vi "Autocompleter.vi"() -> ()   [LabVIEW 2020]
doc: "This VI provides autocomplete suggestions for LabVIEW developers."
uses:
  Model/MarkovModel/MarkovModel.lvclass
  <vilib>/Utility/miscctls.llb/LVBoundsTypeDef.ctl
  <vilib>/Utility/miscctls.llb/LVPositionTypeDef.ctl
  <vilib>/Utility/miscctls.llb/LVPointTypeDef.ctl
panel:
  in  "Stop":bool
  in  "Autowire?":bool
  out "Suggested Block 4":picture caption="Option 4"
  out "Suggested Block 3":picture caption="Option 3"
  out "Suggested Block 2":picture caption="Option 2"
  out "Suggested Block 1":picture caption="Option 1"
  out "Position":T1
  out "Excluded?":bool
  out "Selected":string
  out "value":cluster{"Class Name":string, "Count":i32}[](array[cluster])
  out "One selected?":bool
  out "Active Window":u16(ring) items=["Front Panel", "Block Diagram"]
  out "Selected Object Types":string[](array[string])
  out "Selected VI":string
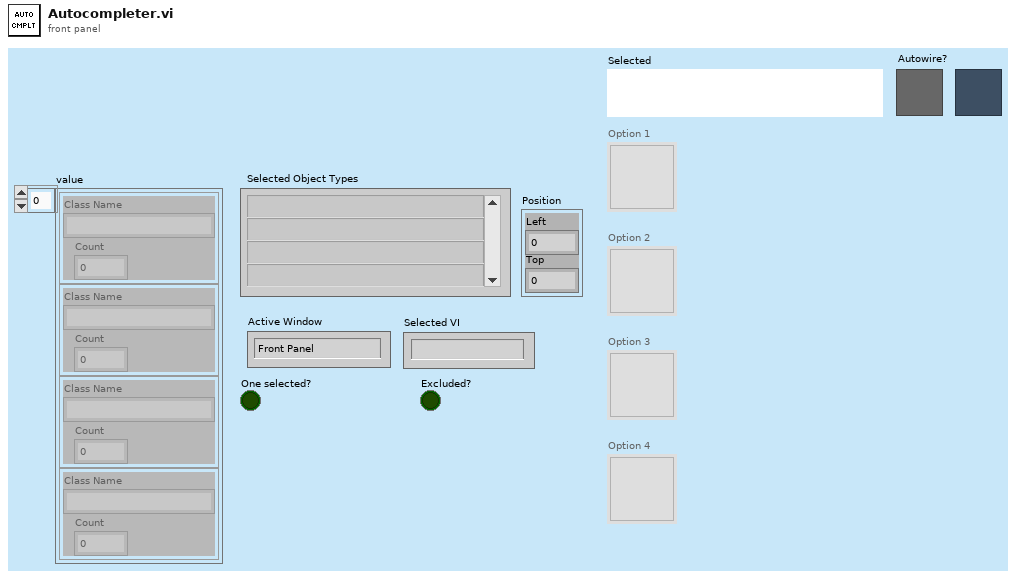
[diagram p1: front panel]
types:
  T1 = typedef "LVPositionTypeDef.ctl" = cluster{"Left":i32, "Top":i32}
  T2 = typedef "LVPointTypeDef.ctl" = cluster{"Horizontal":i16, "Vertical":i16}
  T3 = typedef "imagedata.ctl" = cluster{"image type":i32, "image depth":i32, "image":u8[], "mask":u8[], "colors":u32[], "Rectangle":cluster{"left":i16, "top":i16, "right":i16, "bottom":i16}}
  T4 = enum8{"Enabled", "Disabled", "Disabled and Grayed Out"}
  T5 = typedef "LVBoundsTypeDef.ctl" = cluster{"Width":u32, "Height":u32}
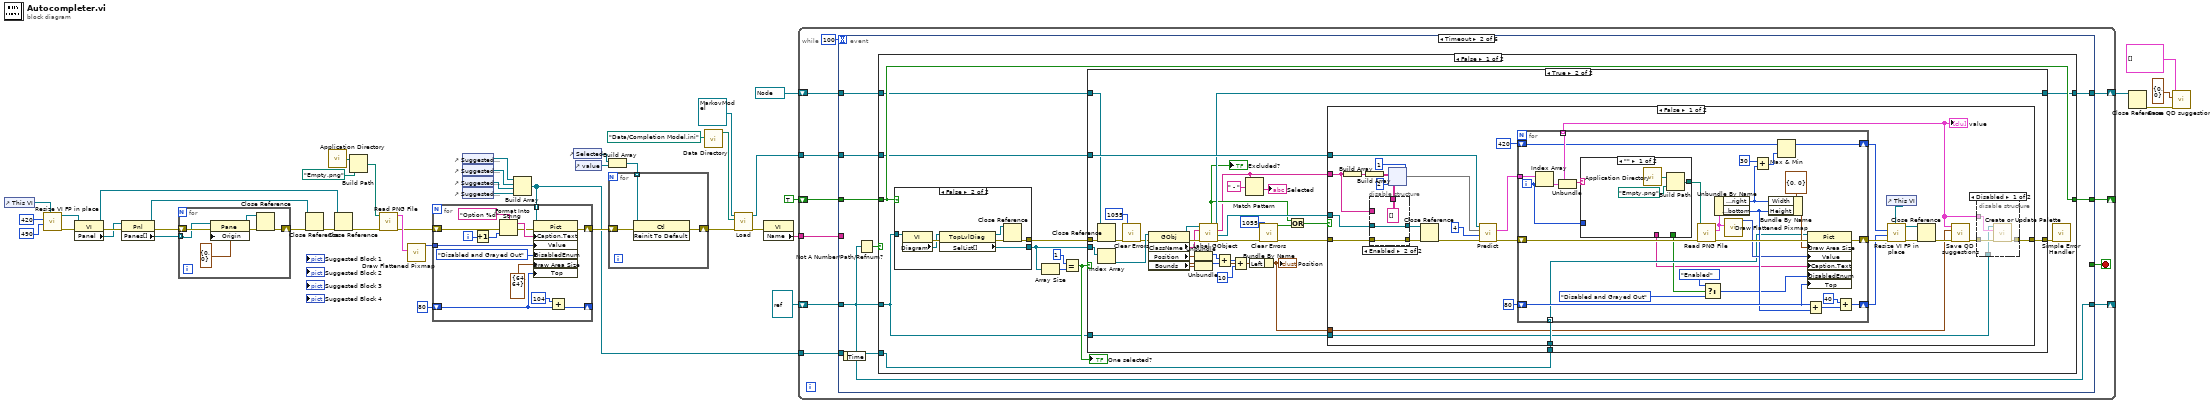
[diagram p0: block diagram]
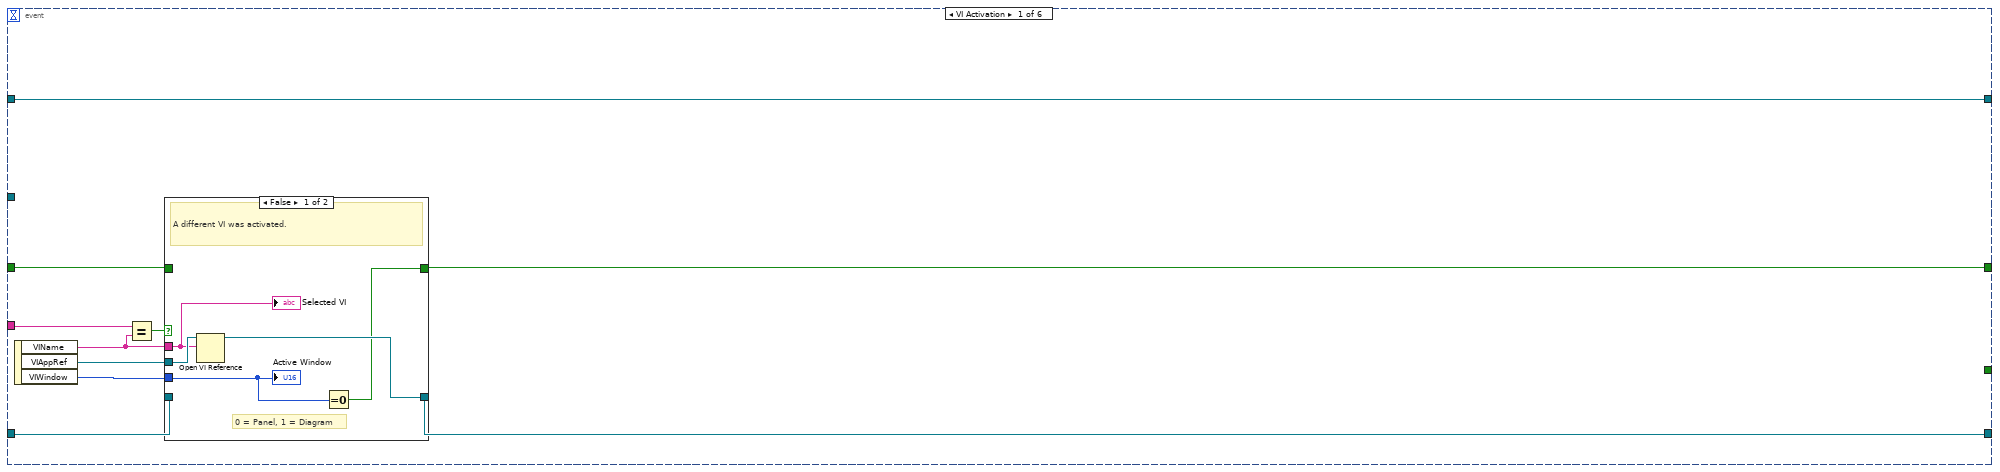
[diagram p2: hidden frame]
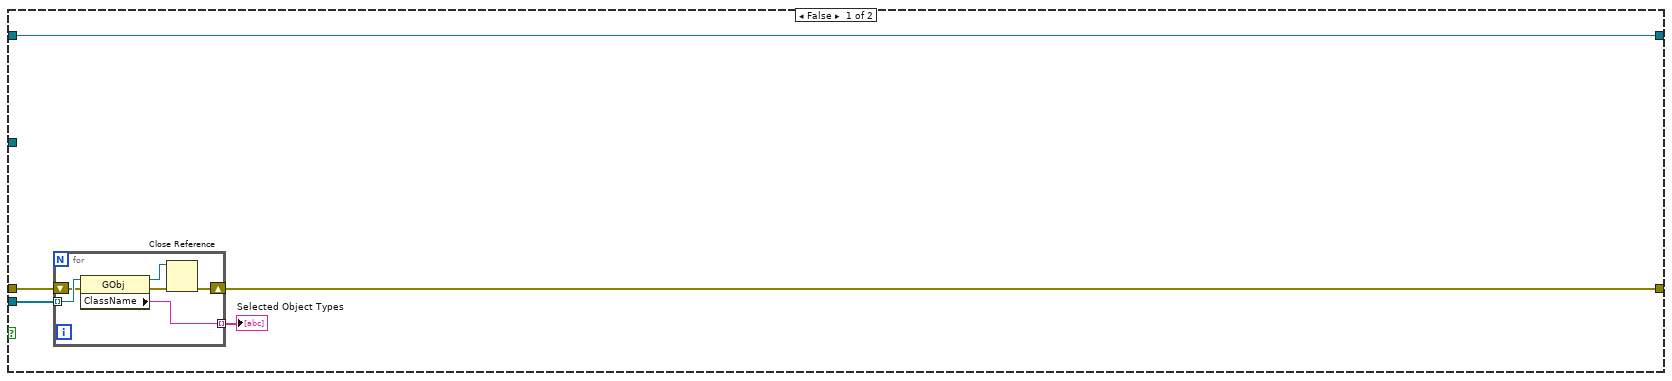
[diagram p4: hidden frame]
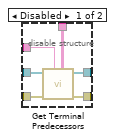
[diagram p6: hidden frame]
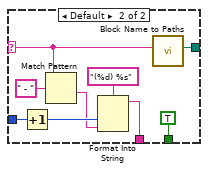
[diagram p7: hidden frame]
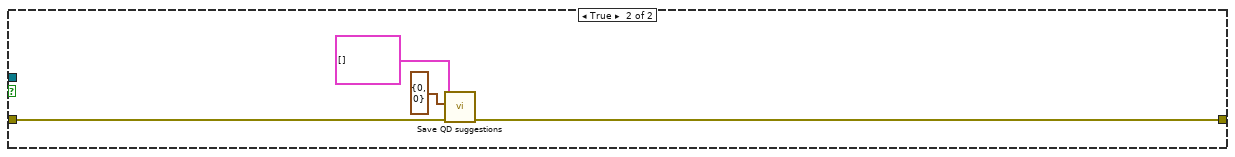
[diagram p8: hidden frame]
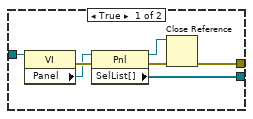
[diagram p9: hidden frame]
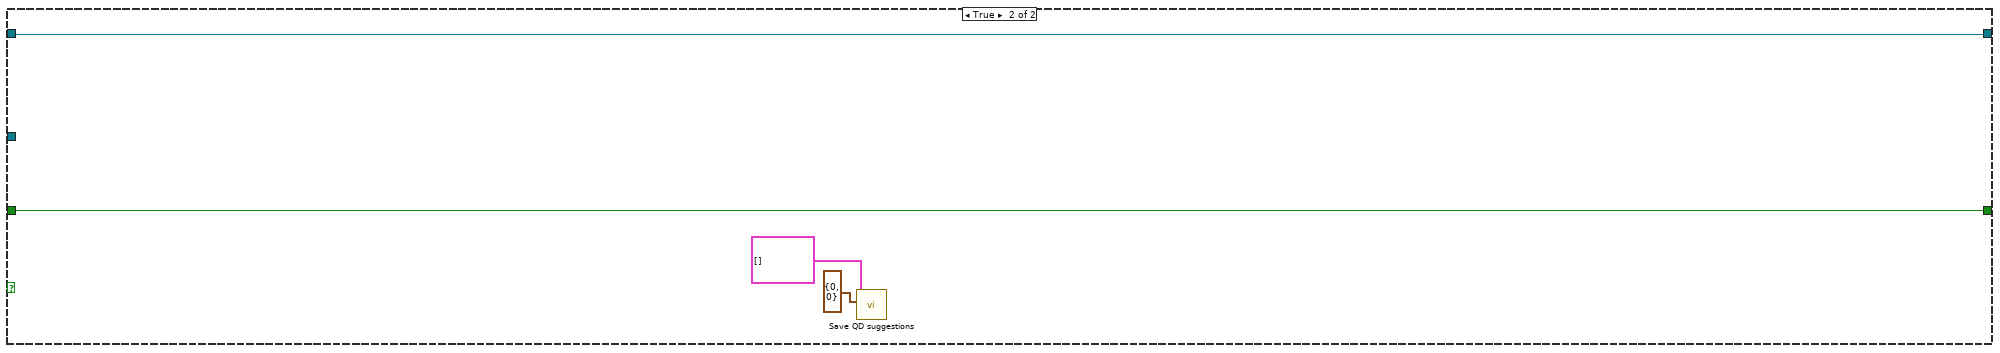
[diagram p10: hidden frame]
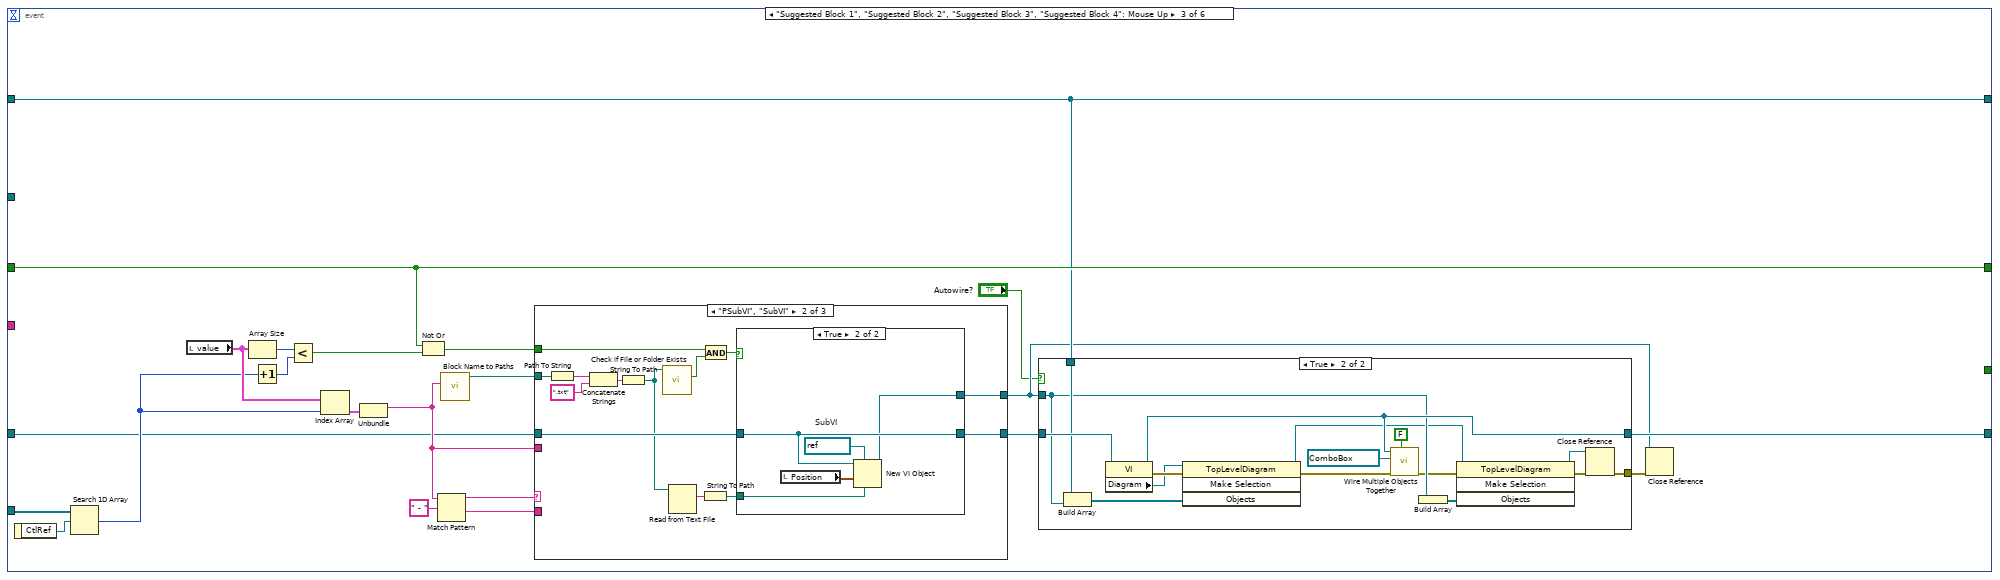
[diagram p11: hidden frame]
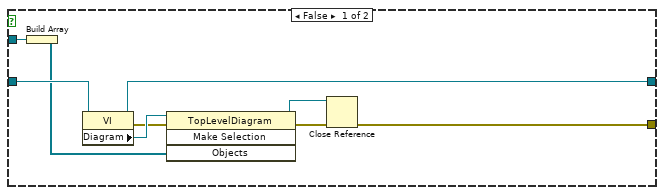
[diagram p12: hidden frame]
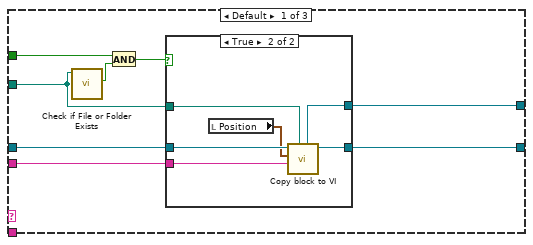
[diagram p13: hidden frame]
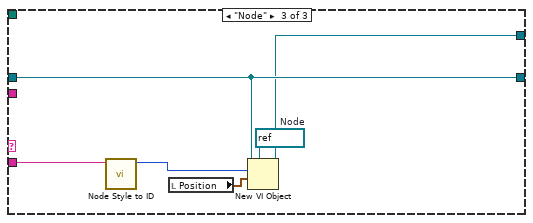
[diagram p16: hidden frame]
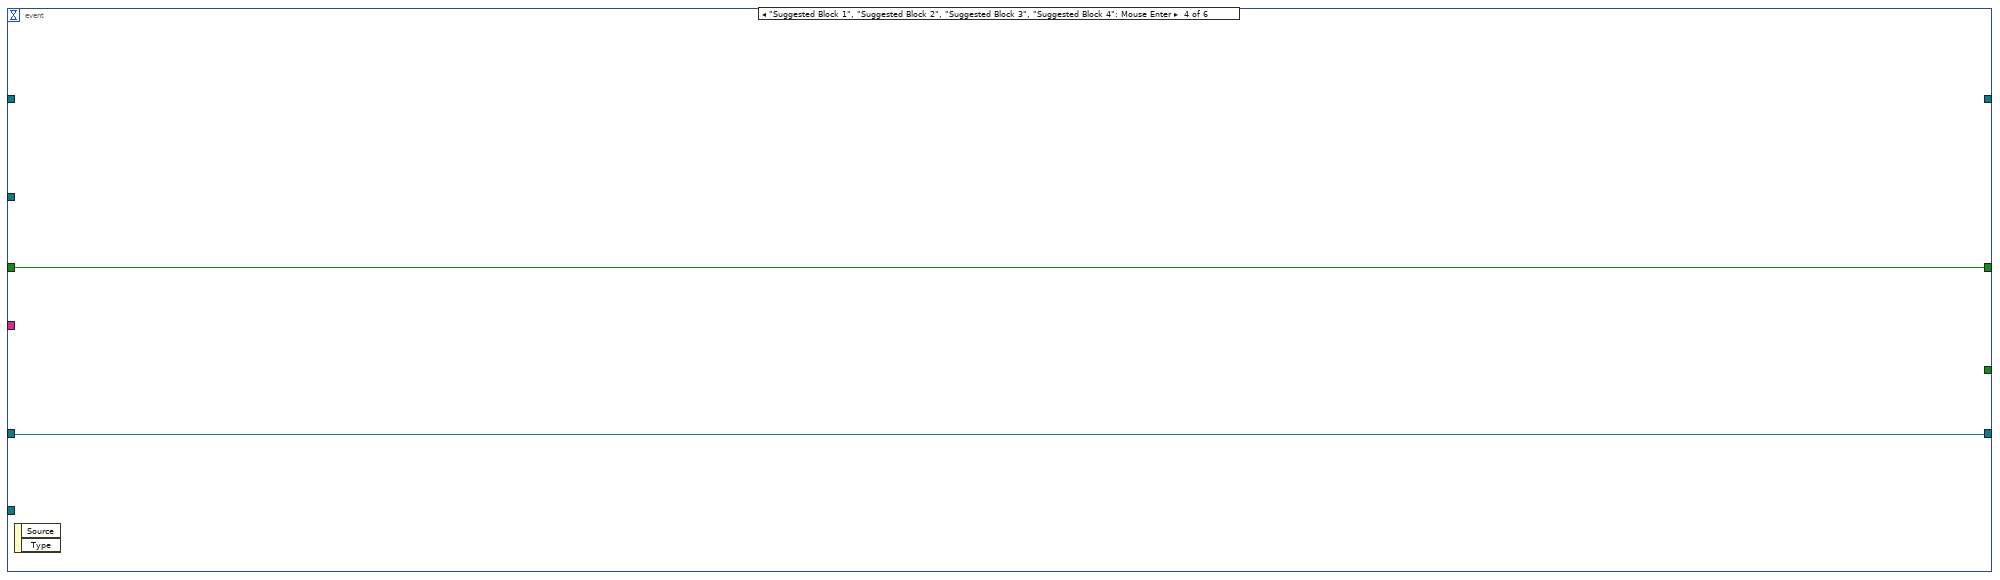
[diagram p17: hidden frame]
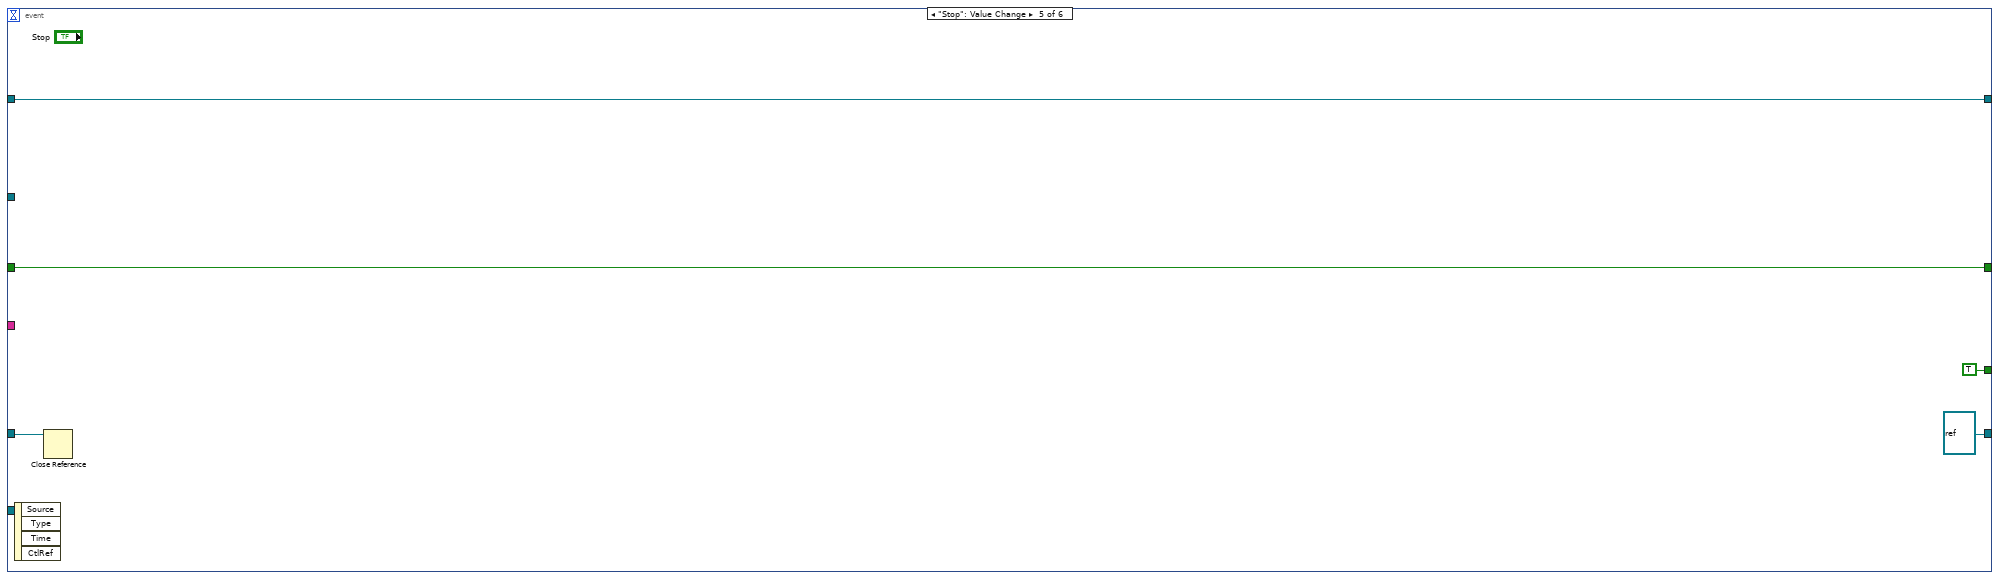
[diagram p18: hidden frame]
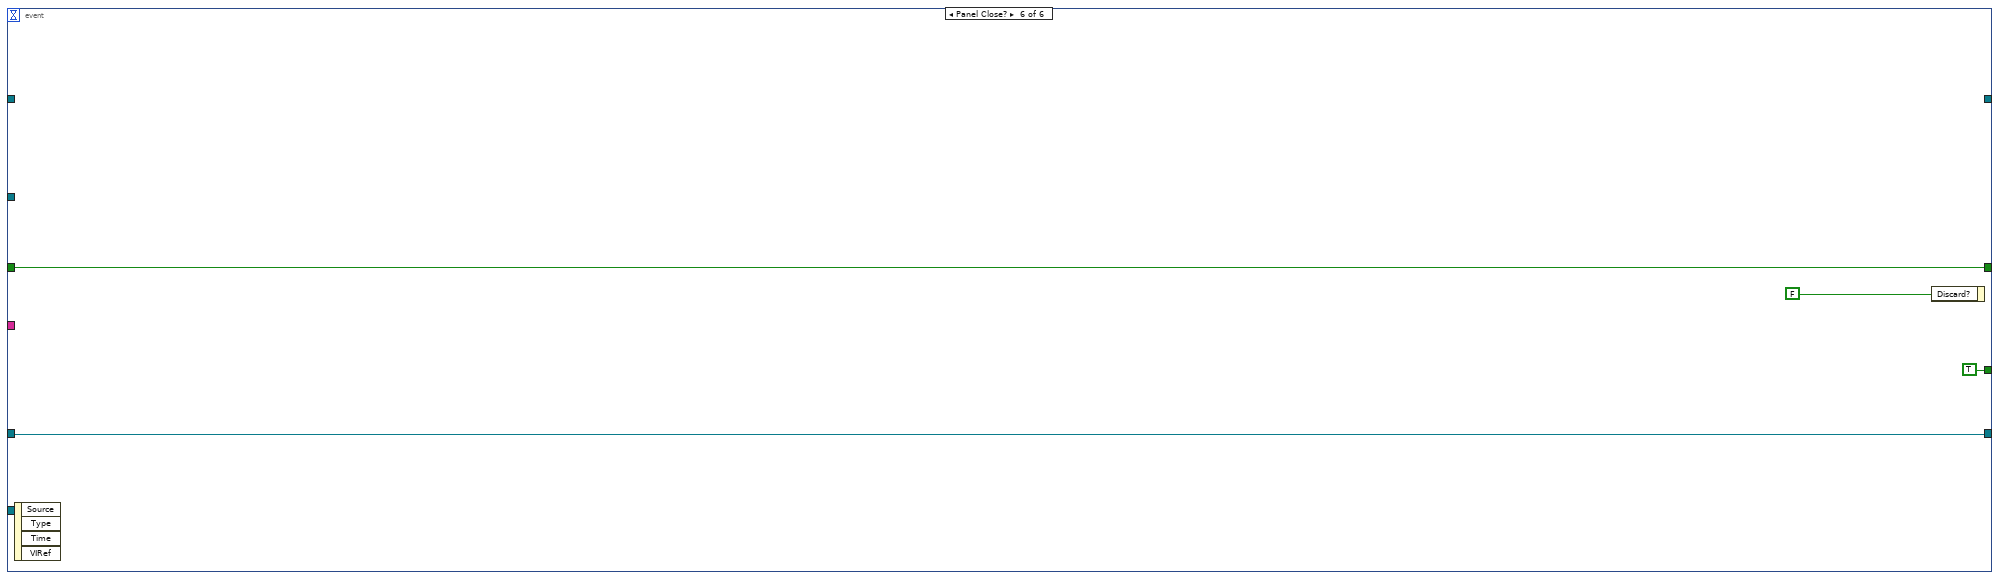
[diagram p19: hidden frame]
diagram:
  n1 = control-ref of="This VI"() -> (w19:refnum<vi>)
  n2 = call "Resize VI FP in place.vi"("VI reference in"=w19, "Height"=u32 490, "Width"=u32 420) -> ("error out"=w11:errorcluster, "VI reference out"=w8:refnum<vi>)  [unwired: 6 in, 1 out]
  n3 = property class="VI"(reference=w8, error in=w11) -> (reference out=w9:refnum<vi>, error out=w16:errorcluster, "Panel"=w7:refnum<vi>)
  n4 = property class="Pnl"(reference=w7, error in=w16) -> (reference out=w13:refnum<vi>, error out=w15:errorcluster, "Panes[]"=w12:refnum<vi>[])
  n5 = for {
    shift-right: [w46] -> w14
    shift-left: w15 -> [w50]
    tunnel: w12 -> [w45] mode=indexing
    n6 = property class="Pane"(reference=w45, error in=w50, "Origin"=T2 {"Horizontal"=0, "Vertical"=0}) -> (reference out=w47:refnum<vi>, error out=w48:errorcluster)
    n7 = Close Reference(reference=w47, error in (no error)=w48) -> (error out=w46:errorcluster)
  }
  n8 = Close Reference(reference=w13, error in (no error)=w14) -> (error out=w10:errorcluster)
  n9 = call <vilib>:"Application Directory.vi"() -> ("Application Directory"=w22:path)
  n10 = Close Reference(reference=w9, error in (no error)=w10) -> (error out=w20:errorcluster)
  n11 = Build Path(base path=w22, name or relative path=path "Empty.png") -> (appended path=w31:path)
  n12 = call <vilib>:"Read PNG File.vi"("error in (no error)"=w20, "path to PNG file"=w31) -> ("error out"=w30:errorcluster, "image data"=w32:T3)  [unwired: 7 in, 1 out]
  n13 = call <vilib>:"Draw Flattened Pixmap.vi"("image data"=w32) -> ("new picture"=w29:picture)  [unwired: 8 in]
  n14 = control-ref of="Suggested Block 1"() -> (w41:refnum<vi>)
  n15 = control-ref of="Suggested Block 2"() -> (w40:refnum<vi>)
  n16 = control-ref of="Suggested Block 3"() -> (w39:refnum<vi>)
  n17 = control-ref of="Suggested Block 4"() -> (w38:refnum<vi>)
  n18 = Build Array(w41, w40, w39, w38) -> (w21:refnum<vi>[])
  n19 = for {
    shift-right: [w64] -> w34
    shift-left: w30 -> [w60]
    tunnel: w21 -> [w63] mode=indexing
    tunnel: w29 -> [w58]
    shift-right: [w55] -> _
    shift-left: 80 -> [w57]
    i -> [w53]
    n20 = Increment(x=w53) -> (x+1=w52:i32)
    n21 = Format Into String(format string="Option %d", error in=w60, w52) -> (resulting string=w61:string, error out=w59:errorcluster)  [unwired: 1 in]
    n22 = property class="Pict"(reference=w63, error in=w59, "Caption.Text"=w61, "Value"=w58, "DisabledEnum"=T4."Disabled and Grayed Out" ("Disabled"), "Draw Area Size"=T5 {"Width"=64, "Height"=64}, "Top"=w57) -> (error out=w64:errorcluster)  [unwired: 1 out]
    n23 = Add(x=104, y=w57) -> (x+y=w55:i32)
  }
  n24 = control-ref of="Selected"() -> (w37:refnum<vi>)
  n25 = control-ref of="value"() -> (w36:refnum<vi>)
  n26 = Build Array(w37, w36) -> (w35:refnum<vi>[])
  n27 = for {
    shift-right: [w67] -> w5
    shift-left: w34 -> [w66]
    tunnel: w35 -> [w65] mode=indexing
    n28 = invoke on="Invoke Node" class="Ctl" method="Reinit To Default"(reference=w65, error in=w66) -> (error out=w67:errorcluster)  [unwired: 1 in, 2 out]
  }
  n29 = call "Data Directory.vi"("Subdirectory"=path "Data/Completion Model.ini" ("file (use dialog)")) -> ("Data directory"=w1:path)  [unwired: 9 in, 1 out]
  n30 = call-dynamic "Load.vi"("error in (no error)"=w5, "Model Path"=w1, "MarkovModel in"=refnum<class "MarkovModel.lvclass"> refnum ("MarkovModel.lvclass")) -> ("error out"=w4:errorcluster, "MarkovModel out"=w2:refnum<class "MarkovModel.lvclass">)  [unwired: 7 in]
  n31 = property class="VI"(error in=w4) -> ("Name"=w44:string)  [unwired: 1 in, 2 out]
  n32 = while {
    tunnel: w44 -> [w77]
    shift-right: [w76] -> _
    shift-left: refnum<vi> refnum ("VIAppRef") -> [w75]
    shift-right: [w72] -> _
    shift-left: TRUE -> [w73]
    tunnel: w2 -> [w71]
    tunnel: w21 -> [w70]
    shift-right: [w68] -> w26
    shift-left: refnum<vi> refnum ("element") -> [w69]
    stop <- w78 stop-if-true
    n33 = event shown="[1] Timeout" {
      selector: _ -> [_ _ _ _ _ _]
      dyn-events: _ -> [_ _ _ _ _ _]
      timeout: 100 -> [_ _ _ _ _ _]
      tunnel: [_ _ _ _ TRUE ("Stop") TRUE ("Stop")] -> w78
      tunnel: w77 -> [w87 _ _ _ _ _]
      tunnel: [w83 w99 w271 w355 refnum<vi> refnum ("VIAppRef") w364] -> w76
      tunnel: w75 -> [w86 w99 w267 w355 w359 w364]
      tunnel: w73 -> [w81 w102 w288 w354 w360 w363]
      tunnel: [w80 w101 w288 w354 w360 w363] -> w72
      tunnel: w71 -> [_ w100 _ _ _ _]
      tunnel: w70 -> [_ w96 w282 _ _ _]
      tunnel: w69 -> [w79 w98 w272 _ w357 _]
      tunnel: [w79 w97 w272 _ w357 _] -> w68
      event VI Activation {
        # "The VI Activation event fires when a VI panel or diagram window becomes active. Use the VIAppRef event data to open a reference to the VI in the correct Application Instance. Store that VI reference in a shift register. The VIWindow event data indicates whether the front panel window or block diagram window was activated. Store this data (as a Boolean) in a shift register as well."
        n34 = event-data() -> ("VIName"=w84:string, "VIAppRef"=w85:refnum<vi>, "VIWindow"=w82:i32)  [unwired: 1 out]
        n35 = Equal?(x=w87, y=w84) -> (x = y?=w88:bool)
        n36 = case shown="False" w88 {
          tunnel: [w90 w95] -> w83
          tunnel: w86 -> [_ w95]
          tunnel: w84 -> [w92 _]
          tunnel: w85 -> [w93 _]
          tunnel: w82 -> [w91 _]
          tunnel: w81 -> [_ w94]
          tunnel: [w89 w94] -> w80
          frame False {
            # "0 = Panel, 1 = Diagram"
            # "A different VI was activated."
            n37 = Open VI Reference(application reference (local)=w93, vi path=w92) -> (vi reference=w90:refnum<vi>)  [unwired: 4 in, 1 out]
            n38 = Equal To 0?(x=w91) -> (x = 0?=w89:bool)
            "Selected VI" <- w92
            "Active Window" <- w91
          }
          frame True {
            # "This VI was activated. Ignore the activation."
          }
        }
      }
      event Timeout {
        # "Use the Timeout case to poll the selection list of the active VI's panel or diagram. Currently, this VI just displays the ClassName property of each selected VI. In your own application that is monitoring active VIs and their selections, you would add your own VI Scripting code in this location."
        n39 = event-data() -> ()  [unwired: 2 out]
        n40 = Not A Number/Path/Refnum?(number/path/refnum=w99) -> (NaN/Path/Refnum?=w103:bool)
        n41 = case shown="False" w103 {
          tunnel: w102 -> [w115 w266]
          tunnel: w99 -> [w104 _]
          tunnel: [w115 w266] -> w101
          tunnel: w100 -> [w108 _]
          tunnel: w98 -> [w107 w265]
          tunnel: [w106 w265] -> w97
          tunnel: w96 -> [w105 _]
          frame False {
            n42 = case shown="False" w115 {
              tunnel: [w253 w261] -> w111
              tunnel: [w251 w259] -> w110
              tunnel: w104 -> [w249 w257]
              frame True {
                n43 = property class="VI"(reference=w249) -> (error out=w255:errorcluster, "Panel"=w254:refnum<vi>)  [unwired: 1 in, 1 out]
                n44 = property class="Pnl"(reference=w254, error in=w255) -> (reference out=w250:refnum<vi>, error out=w252:errorcluster, "SelList[]"=w253:refnum<vi>[])
                n45 = Close Reference(reference=w250, error in (no error)=w252) -> (error out=w251:errorcluster)
              }
              frame False {
                n46 = property class="VI"(reference=w257) -> (error out=w262:errorcluster, "Diagram"=w256:refnum<vi>)  [unwired: 1 in, 1 out]
                n47 = property class="TopLvlDiag"(reference=w256, error in=w262) -> (reference out=w258:refnum<vi>, error out=w260:errorcluster, "SelList[]"=w261:refnum<vi>[])
                n48 = Close Reference(reference=w258, error in (no error)=w260) -> (error out=w259:errorcluster)
              }
            }
            n49 = Array Size(array=w111) -> (size(s)=w114:i32)
            n50 = Equal?(x=1, y=w114) -> (x = y?=w112:bool)
            "One selected?" <- w112
            n51 = case shown="True" w112 {
              tunnel: w111 -> [w119 w159]
              tunnel: w110 -> [w118 w144]
              tunnel: [w116 w156] -> w109
              tunnel: w108 -> [_ w155]
              tunnel: w107 -> [w117 w143]
              tunnel: [w117 w137] -> w106
              tunnel: w105 -> [_ w139]
              tunnel: w104 -> [_ w136]
              frame False {
                n52 = for {
                  tunnel: w119 -> [w126] mode=indexing
                  tunnel: [w124] -> w120 mode=indexing
                  shift-right: [w122] -> w116
                  shift-left: w118 -> [w125]
                  n53 = property class="GObj"(reference=w126, error in=w125) -> (reference out=w121:refnum<vi>, error out=w123:errorcluster, "ClassName"=w124:string)
                  n54 = Close Reference(reference=w121, error in (no error)=w123) -> (error out=w122:errorcluster)
                }
                "Selected Object Types" <- w120
              }
              frame True {
                n55 = Close Reference(reference=w143, error in (no error)=w144) -> (error out=w142:errorcluster)
                n56 = Index Array(array=w159) -> (element=w145:refnum<vi>)  [unwired: 1 in]
                n57 = call <vilib>:"Clear Errors.vi"("error in (no error)"=w142, "specific error code to clear (0: all)"=1055) -> ("error out"=w141:errorcluster)  [unwired: 4 in, 1 out]
                n58 = property class="GObj"(reference=w145, error in=w141) -> (reference out=w147:refnum<vi>, error out=w158:errorcluster, "ClassName"=w157:string, "Position"=w149:T1, "Bounds"=w154:T5)
                n59 = Unbundle(w149) -> ("Left"=w153:i32)  [unwired: 1 out]
                n60 = Unbundle(w154) -> ("Width"=w152:u32)  [unwired: 1 out]
                n61 = call "Label GObject.vi"("error in"=w158, "GObject ClassName"=w157, "GObject Reference In"=w147) -> ("error out"=w134:errorcluster, "Terminals[]"=w146:refnum<vi>[], "Label"=w127:string, "GObject Reference out"=w137:refnum<vi>, "Excluded?"=w131:bool)  [unwired: 4 in]
                "Excluded?" <- w131
                n62 = Add(x=w153, y=w152) -> (x+y=w151:u32)
                n63 = Add(x=w151, y=u32 10) -> (x+y=w148:u32)
                n64 = Match Pattern(string=w127, regular expression=" - ") -> (after substring=→"Selected":string)  [unwired: 1 in, 3 out]
                n65 = Bundle By Name(cluster=w149, "Left"=w148) -> (w138:T1)
                "Position" <- w138
                n66 = call <vilib>:"Clear Errors.vi"("error in (no error)"=w134, "specific error code to clear (0: all)"=1055) -> ("error out"=w133:errorcluster, "specific error cleared?"=w132:bool)  [unwired: 4 in]
                n67 = Or(x=w131, y=w132) -> (x .or. y?=w130:bool)
                n68 = case shown="False" w130 {
                  tunnel: w133 -> [w188 w247]
                  tunnel: [w171 w248] -> w156
                  tunnel: w127 -> [w186 _]
                  tunnel: w155 -> [w163 _]
                  tunnel: w146 -> [w187 _]
                  tunnel: w139 -> [w169 _]
                  tunnel: w138 -> [w167 _]
                  tunnel: w136 -> [w166 _]
                  frame False {
                    n69 = Build Array(w186) -> (w183:string[])
                    n70 = Build Array(w183) -> (w182:string[][])
                    n71 = disable-structure shown="Enabled" {
                      disable-tunnel: [w201 w203] -> w190
                      disable-tunnel: [w200 w204] -> w189
                      disable-tunnel: w188 -> [w199 w203]
                      disable-tunnel: w187 -> [w198 w204]
                      disable-tunnel: w186 -> [w197 _]
                      disable-tunnel: [w196 string[][] [] ("2nd Order Queries")] -> w181
                      frame Disabled {
                        n72 = call "Get Terminal Predecessors.vi"("Selected"=w197, "error in (no error)"=w199, "Terminals[] in"=w198) -> ("error out"=w201:errorcluster, "Terminals[] out"=w200:refnum<vi>[], "2nd Order Queries"=w196:string[][])  [unwired: 6 in]
                      }
                      frame Enabled {
                      }
                    }
                    n73 = node(1, w182, 2 ("key"), w181) -> (w162:map{i32, string[][]})
                    n74 = Close Reference(reference=w189, error in (no error)=w190) -> (error out=w165:errorcluster)
                    n75 = call-dynamic "Predict.vi"("error in (no error)"=w165, "Length"=4 ("length"), "Candidate Map"=w162, "MarkovModel in"=w163) -> ("error out"=w164:errorcluster, "Winners"=w160:cluster{"Class Name":string, "Count":i32}[])  [unwired: 5 in, 1 out]
                    n76 = for {
                      shift-right: [w229] -> w178
                      shift-left: w164 -> [w232]
                      tunnel: w160 -> [w221]
                      tunnel: [w220] -> w170 mode=indexing
                      shift-right: [w223] -> w175
                      shift-left: 80 -> [w226]
                      shift-right: [w213] -> w176
                      shift-left: 420 ("Numeric") -> [w214]
                      tunnel: w169 -> [w208] mode=indexing
                      i -> [w205]
                      n77 = Index Array(array=w221, index=w205) -> (element=w220:cluster{"Class Name":string, "Count":i32})
                      n78 = Unbundle(w220) -> ("Class Name"=w219:string)  [unwired: 1 out]
                      n79 = case shown="\"\"" w219 {
                        selector: w219 -> [_ w237]
                        tunnel: [w234 w244] -> w231
                        tunnel: [_ TRUE ("Visible")] -> w207
                        tunnel: [_ w241] -> w206
                        tunnel: w205 -> [_ w239]
                        frame "" {
                          n80 = call <vilib>:"Application Directory.vi"() -> ("Application Directory"=w233:path)
                          n81 = Build Path(base path=w233, name or relative path=path "Empty.png") -> (appended path=w234:path)
                        }
                        frame Default {
                          n82 = Increment(x=w239) -> (x+1=w240:i32)
                          n83 = Match Pattern(string=w237, regular expression=" - ") -> (after substring=w236:string)  [unwired: 1 in, 3 out]
                          n84 = Format Into String(format string="(%d) %s", w240, w236) -> (resulting string=w241:string)  [unwired: 2 in, 1 out]
                          n85 = call "Block Name to Paths.vi"("Block Name"=w237) -> ("Image Path"=w244:path)  [unwired: 9 in, 1 out]
                        }
                      }
                      n86 = call <vilib>:"Read PNG File.vi"("error in (no error)"=w232, "path to PNG file"=w231) -> ("error out"=w230:errorcluster, "image data"=w228:T3)  [unwired: 7 in, 1 out]
                      n87 = Select(t=T4."Enabled" ("Disabled"), s=w207, f=T4."Disabled and Grayed Out" ("Disabled")) -> (s? t:f=w217:T4)
                      n88 = Unbundle By Name(w228) -> ("Rectangle.right"=w212:i16, "Rectangle.bottom"=w225:i16)
                      n89 = call <vilib>:"Draw Flattened Pixmap.vi"("image data"=w228) -> ("new picture"=w216:picture)  [unwired: 8 in]
                      n90 = Add(x=i16 30, y=w212) -> (x+y=w211:i16)
                      n91 = Bundle By Name(cluster=T5 {"Width"=0, "Height"=0} ("Draw Area Size"), "Width"=w212, "Height"=w225) -> (w215:T5)
                      n92 = Max & Min(x=w214, y=w211) -> (max(x,y)=w213:i32)  [unwired: 1 out]
                      n93 = Add(x=w226, y=w225) -> (x+y=w224:i32)
                      n94 = property class="Pict"(reference=w208, error in=w230, "Draw Area Size"=w215, "Value"=w216, "Caption.Text"=w206, "DisabledEnum"=w217, "Top"=w226) -> (error out=w229:errorcluster)  [unwired: 1 out]
                      n95 = Add(x=40, y=w224) -> (x+y=w223:i32)
                    }
                    "value" <- w170
                    n96 = control-ref of="This VI"() -> (w168:refnum<vi>)
                    n97 = call "Resize VI FP in place.vi"("VI reference in"=w168, "error in (no error)"=w178, "Height"=w175, "Width"=w176) -> ("error out"=w177:errorcluster, "VI reference out"=w174:refnum<vi>)  [unwired: 5 in, 1 out]
                    n98 = Close Reference(reference=w174, error in (no error)=w177) -> (error out=w173:errorcluster)
                    n99 = call "Save QD suggestions.vi"("error in"=w173, "Position"=w167, "Suggestions"=w170) -> ("error out"=w172:errorcluster)  [unwired: 8 in]
                    n100 = disable-structure shown="Disabled" {
                      disable-tunnel: w172 -> [w194 w195]
                      disable-tunnel: [w193 w195] -> w171
                      disable-tunnel: w170 -> [w192 _]
                      disable-tunnel: w166 -> [w191 _]
                      frame Disabled {
                        n101 = call "Create or Update Palette.vi"("error in (no error)"=w194, "Suggestions"=w192, "VIAppRef"=w191) -> ("error out"=w193:errorcluster)  [unwired: 7 in, 1 out]
                      }
                      frame Enabled {
                      }
                    }
                  }
                  frame True {
                    n102 = call "Save QD suggestions.vi"("error in"=w247, "Position"=T1 {"Left"=0, "Top"=0}, "Suggestions"=cluster{"Class Name":string, "Count":i32}[] []) -> ("error out"=w248:errorcluster)  [unwired: 8 in]
                  }
                }
              }
            }
            n103 = call <vilib>:"Simple Error Handler.vi"("error in (no error)"=w109) -> ()  [unwired: 4 in, 5 out]
          }
          frame True {
            n104 = call "Save QD suggestions.vi"("Position"=T1 {"Left"=0, "Top"=0}, "Suggestions"=cluster{"Class Name":string, "Count":i32}[] []) -> ()  [unwired: 9 in, 1 out]
          }
        }
      }
      event "Suggested Block 1", "Suggested Block 2", "Suggested Block 3", "Suggested Block 4": Mouse Up {
        n105 = event-data() -> ("CtlRef"=w275:refnum<vi>)  [unwired: 1 out]
        n106 = Search 1D Array(1D array=w282, element=w275) -> (index of element=w280:i32)  [unwired: 1 in]
        n107 = local read "value"() -> (w285:cluster{"Class Name":string, "Count":i32}[])
        n108 = Array Size(array=w285) -> (size(s)=w284:i32)
        n109 = Increment(x=w280) -> (x+1=w281:i32)
        n110 = Less?(x=w284, y=w281) -> (x < y?=w283:bool)
        n111 = Index Array(array=w285, index=w280) -> (element=w287:cluster{"Class Name":string, "Count":i32})
        n112 = Unbundle(w287) -> ("Class Name"=w277:string)  [unwired: 1 out]
        n113 = Not Or(1:w283, 2:w288) -> (0:w286:bool)
        n114 = Match Pattern(string=w277, regular expression=" - ") -> (before substring=w276:string, after substring=w274:string)  [unwired: 1 in, 2 out]
        n115 = call "Block Name to Paths.vi"("Block Name"=w277) -> ("Block Path"=w279:path)  [unwired: 9 in, 1 out]
        n116 = case shown="\"PSubVI\", \"SubVI\"" w276 {
          tunnel: w286 -> [w321 w341 _]
          tunnel: w267 -> [w318 w338 w351]
          tunnel: [w317 w337 w351] -> w273
          tunnel: w277 -> [w316 _ _]
          tunnel: w279 -> [w315 w336 _]
          tunnel: w274 -> [_ _ w349]
          tunnel: [w314 w329 w350] -> w269
          frame Default {
            n117 = call <vilib>:"Check if File or Folder Exists.vi"("path"=w315) -> ("file or folder exists?"=w320:bool)  [unwired: 8 in, 2 out]
            n118 = And(x=w321, y=w320) -> (x .and. y?=w319:bool)
            n119 = case shown="True" w319 {
              tunnel: w315 -> [_ w328]
              tunnel: w318 -> [w322 w327]
              tunnel: [w322 w326] -> w317
              tunnel: w316 -> [_ w325]
              tunnel: [_ w323] -> w314
              frame False {
              }
              frame True {
                n120 = local read "Position"() -> (w324:T1)
                n121 = call "Copy block to VI.vi"("Block path"=w328, "Object Label"=w325, "position"=w324, "Target VI reference in"=w327) -> ("Target VI reference out"=w326:refnum<vi>, "GObject reference out"=w323:refnum<vi>)  [unwired: 5 in, 1 out]
              }
            }
          }
          frame "PSubVI", "SubVI" {
            n122 = Path To String(path=w336) -> (string=w335:string)
            n123 = Concatenate Strings(w335, ".txt" ("string")) -> (w333:string)
            n124 = String To Path(string=w333) -> (path=w332:path)
            n125 = call <vilib>:"Check if File or Folder Exists.vi"("path"=w332) -> ("file or folder exists?"=w340:bool)  [unwired: 8 in, 2 out]
            n126 = Read from Text File(file (use dialog)=w332) -> (text=w331:string)  [unwired: 3 in, 3 out]
            n127 = String To Path(string=w331) -> (path=w330:path)
            n128 = And(x=w341, y=w340) -> (x .and. y?=w339:bool)
            n129 = case shown="True" w339 {
              tunnel: w338 -> [w342 w345]
              tunnel: [w342 w345] -> w337
              tunnel: w330 -> [_ w344]
              tunnel: [_ w343] -> w329
              frame False {
              }
              frame True {
                w347 = refnum<vi> refnum  # SubVI
                n130 = local read "Position"() -> (w346:T1)
                n131 = New VI Object(vi object class=w347, owner refnum=w345, position/next to=w346, 6:w344) -> (object refnum=w343:refnum<vi>)  [unwired: 4 in, 1 out]
              }
            }
          }
          frame "Node" {
            w352 = refnum<vi> refnum  # Node
            n132 = call "Node Style to ID.vi"("Function Name"=w349) -> ("Function ID"=w348:i32)  [unwired: 9 in, 1 out]
            n133 = local read "Position"() -> (w353:T1)
            n134 = New VI Object(vi object class=w352, owner refnum=w351, style=w348, position/next to=w353) -> (object refnum=w350:refnum<vi>)  [unwired: 4 in, 1 out]
          }
        }
        n135 = case shown="True" "Autowire?" {
          tunnel: w273 -> [w294 w313]
          tunnel: w272 -> [_ w312]
          tunnel: [w295 w311] -> w271
          tunnel: [w291 w308] -> w270
          tunnel: w269 -> [w290 w307]
          frame False {
            n136 = Build Array(w290) -> (w289:refnum<vi>[])
            n137 = property class="VI"(reference=w294) -> (reference out=w295:refnum<vi>, error out=w296:errorcluster, "Diagram"=w297:refnum<vi>)  [unwired: 1 in]
            n138 = invoke class="TopLevelDiagram" method="Make Selection"(reference=w297, error in=w296, "Objects"=w289) -> (reference out=w292:refnum<vi>, error out=w293:errorcluster)  [unwired: 1 in, 2 out]
            n139 = Close Reference(reference=w292, error in (no error)=w293) -> (error out=w291:errorcluster)
          }
          frame True {
            n140 = Build Array(w312, w307) -> (w303:refnum<vi>[])
            n141 = property class="VI"(reference=w313) -> (reference out=w311:refnum<vi>, error out=w306:errorcluster, "Diagram"=w305:refnum<vi>)  [unwired: 1 in]
            n142 = invoke class="TopLevelDiagram" method="Make Selection"(reference=w305, error in=w306, "Objects"=w303) -> (reference out=w298:refnum<vi>, error out=w304:errorcluster)  [unwired: 1 in, 2 out]
            n143 = call <resource>:"Wire Multiple Objects Together.vi"("Shift Pressed?"=FALSE, "error in (no error)"=w304, "QD Combo Box Ref"=refnum<vi> refnum, "QD Launch VI Ref"=w311) -> ("error out"=w300:errorcluster)  [unwired: 6 in, 1 out]
            n144 = Build Array(w307) -> (w299:refnum<vi>[])
            n145 = invoke class="TopLevelDiagram" method="Make Selection"(reference=w298, error in=w300, "Objects"=w299) -> (reference out=w309:refnum<vi>, error out=w310:errorcluster)  [unwired: 1 in, 2 out]
            n146 = Close Reference(reference=w309, error in (no error)=w310) -> (error out=w308:errorcluster)
          }
        }
        n147 = Close Reference(reference=w269, error in (no error)=w270) -> ()  [unwired: 1 out]
      }
      event "Suggested Block 1", "Suggested Block 2", "Suggested Block 3", "Suggested Block 4": Mouse Enter {
        n148 = event-data() -> ()  [unwired: 3 out]
      }
      event "Stop": Value Change {
        # "Stop the VI and close the stored VI reference."
        n149 = event-data() -> ()  [unwired: 5 out]
        n150 = Close Reference(reference=w359) -> ()  [unwired: 1 in, 1 out]
      }
      event Panel Close? {
        n151 = event-data() -> ()  [unwired: 5 out]
        n152 = event-data("Discard?"=FALSE) -> ()  [unwired: 1 in, 1 out]
      }
    }
  }
  n153 = Close Reference(reference=w26) -> (error out=w23:errorcluster)  [unwired: 1 in]
  n154 = call "Save QD suggestions.vi"("error in"=w23, "Position"=T1 {"Left"=0, "Top"=0}, "Suggestions"=cluster{"Class Name":string, "Count":i32}[] []) -> ()  [unwired: 8 in, 1 out]
